vi "Start Menu.vi"(5 "Stats":string[][](table) caption="Result Set (from first statement with results)", 7 "Data Out":string[][](table) caption="Result Set (from first statement with results)", 8 "error in (no error)":errorcluster, 11 "Enum":enum16{"Initial Menu", "Final Menu"}(ring)) -> (0 "error out":errorcluster, 3 "Start/Stop":bool)   [LabVIEW 2021, in "Board Game.lvlib"]
uses:
  Board Game.lvlib
  <vilib>/Utility/miscctls.llb/LVRowAndColumnTypeDef.ctl
  Modules/Sound Manager/Typedefs/Sound Effects.ctl
  Utilities/Globales Snake.vi
  Modules/Sound Manager/Sound Manager.lvlib
panel:
  out "GAME STATS":bool
  in  "Player Name":string="user"
  out "INSTRUCTIONS":bool
  in  "Start Game":bool
  in  "GAME STATS":i32(listbox)
  out "LEADERBOARD":bool
  out "Instructions":bool
  in  "Play/stop":bool
  in  "Stop":bool
  in  "LEADERBOARD":i32(listbox)
  in  "Number of Bombs":i32=1
  in  "Play with Bombs":bool
  in  "Music:":u32(ring) items=["Music 1", "Music 2", "Music 3", "Music 4"]
  in  "Game Difficulty:":u32(ring)=150 items=["Easy"=750, "Hard"=500, "Extreme"=300, "Carlo Music"=150]
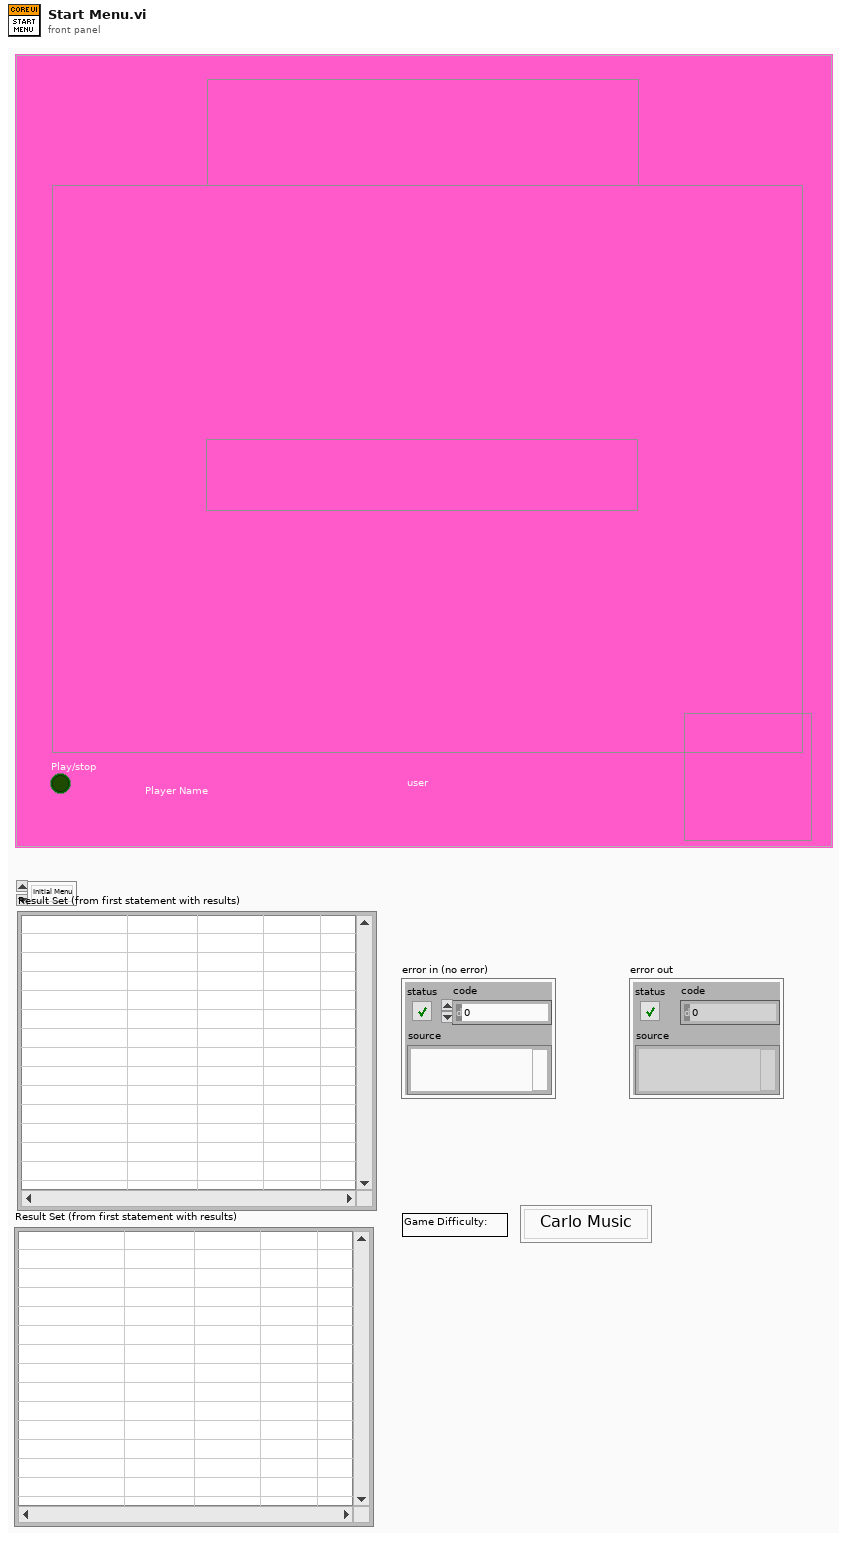
[diagram p1: front panel]
types:
  T1 = typedef "Sound Manager.lvlib/Sound Effects.ctl" = enum16{"Bomb In", "Bomb Out", "Bomb Touched", "Game Over", "Victory", "Eat", "10 Fruits", "Eat2", "Eat3", "Eat4", "MaxShield", "Shield", "10p", "Grape In", "Grape Out", "20p", "30p", "40p", "50p", "60p", "70p", "80p", "90p", "100p", "All shields cracked", "Mouse In", "Mouse Out", "Mouse Eaten", "Grape Eaten", "States Recover", "Broken Shield", "Bonus", "Happy Time", "explode", "Game over musica", "Back Music", "Shield Catch", "Evil lough", "Cricket In", "Cricket eaten", "Lets Go", "Jump1", "Jump2", "Jump3", "Unstoppable", "Troll Music", "winner", "menu"}
  T2 = typedef "LVRowAndColumnTypeDef.ctl" = cluster{"Row":i32, "Column":i32}
  T3 = cluster{"Music:":u32, "Game Difficulty:":u32, "Number of Bombs":i32}
  T4 = enum32{"Invalid", "Standard", "Closed", "Hidden", "Minimized", "Maximized"}
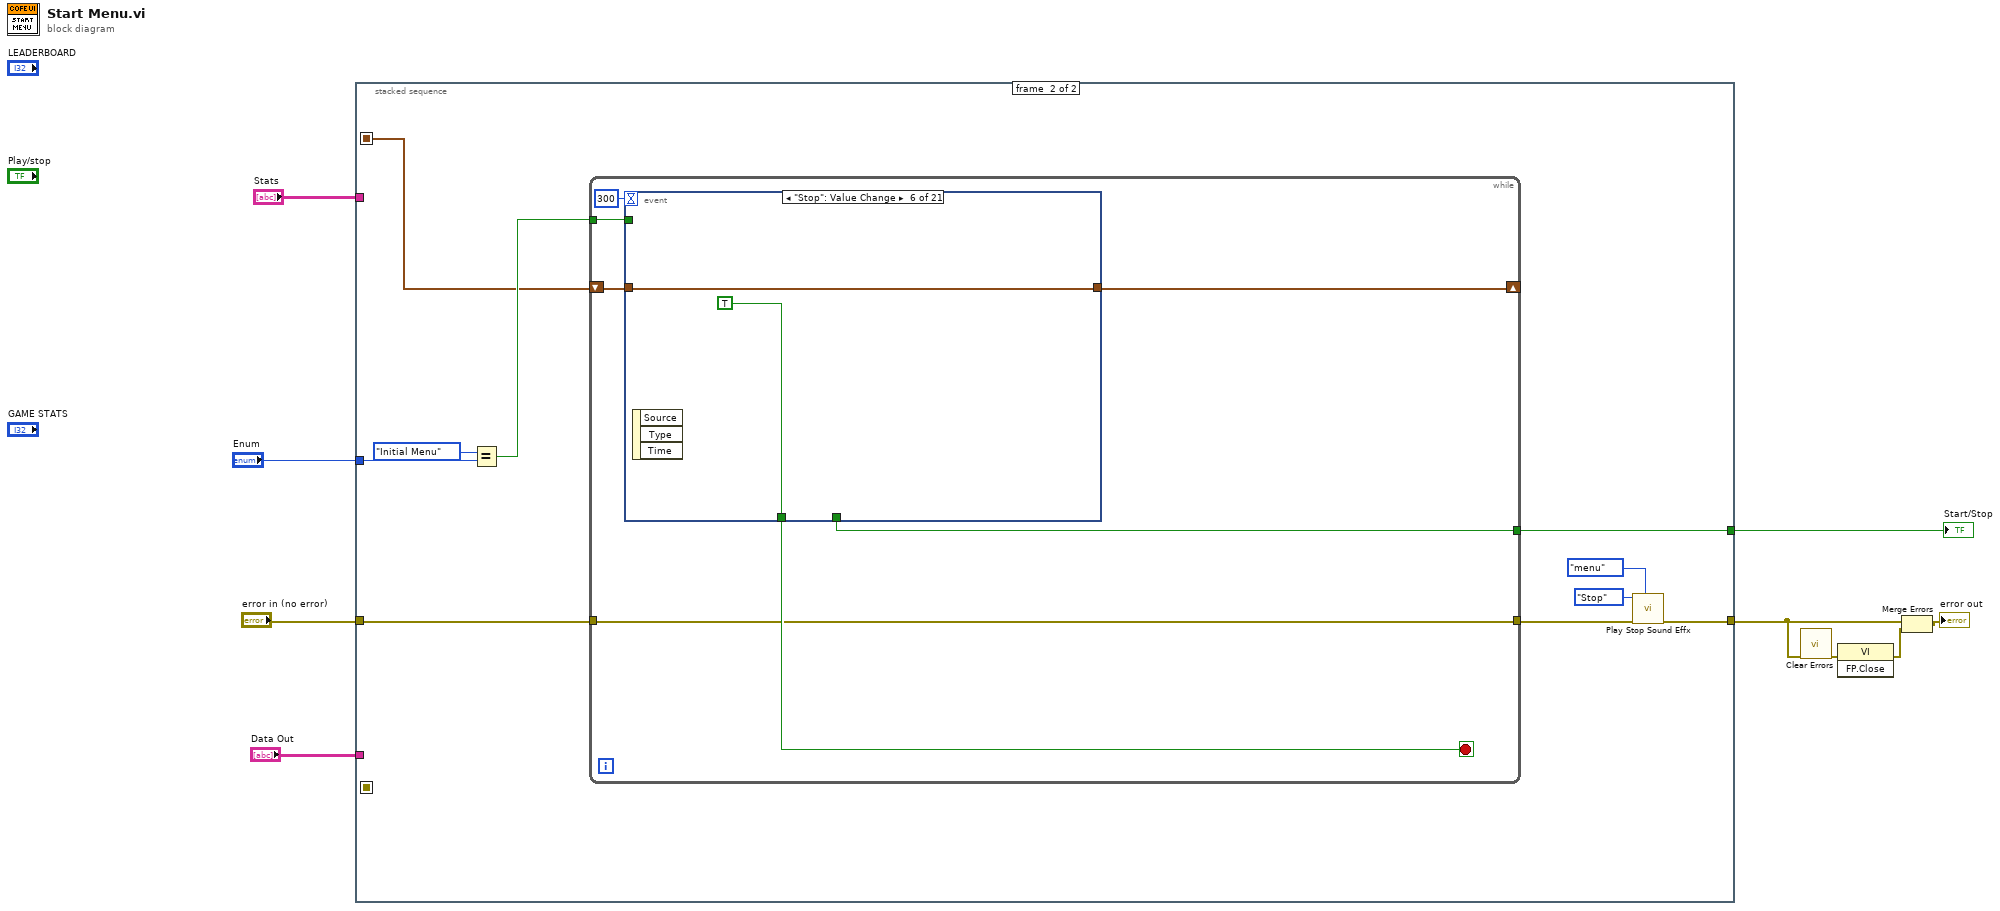
[diagram p0: block diagram]
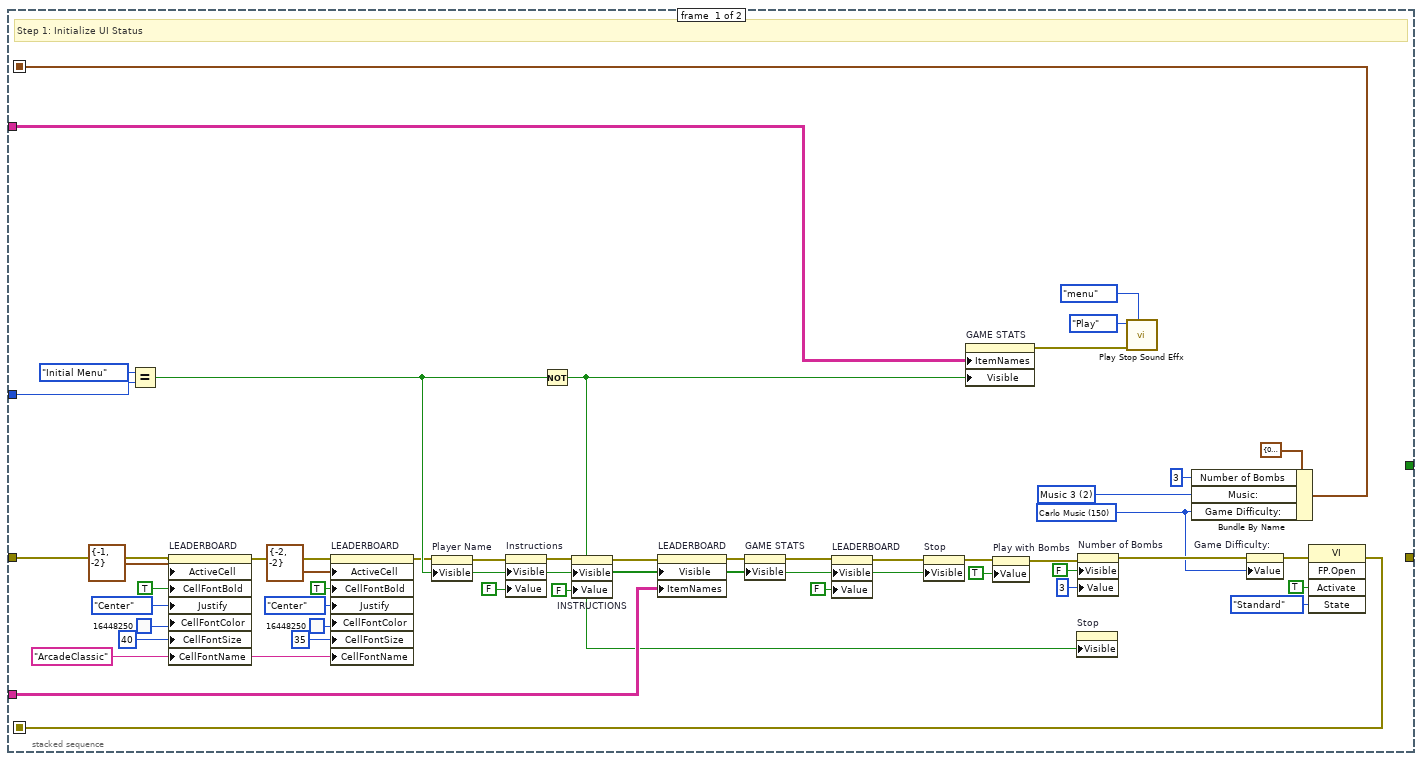
[diagram p2: hidden frame]
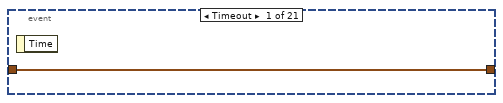
[diagram p3: hidden frame]
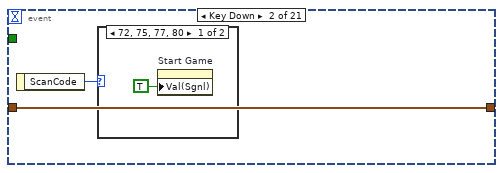
[diagram p4: hidden frame]
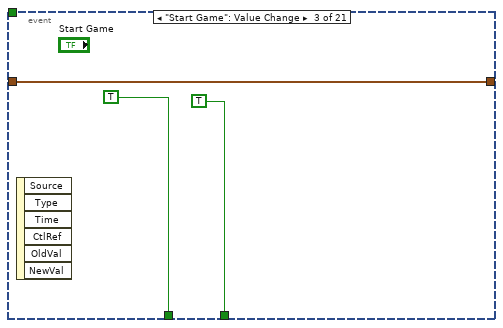
[diagram p6: hidden frame]
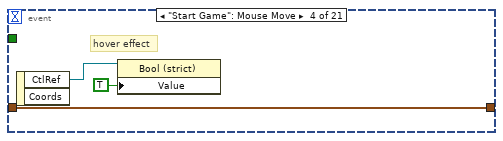
[diagram p7: hidden frame]
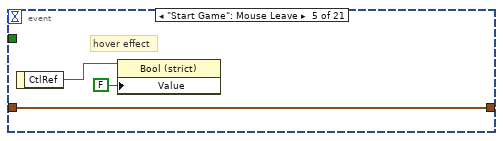
[diagram p8: hidden frame]
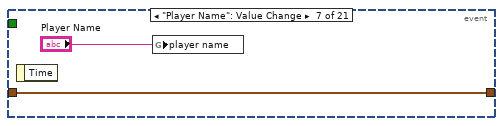
[diagram p9: hidden frame]
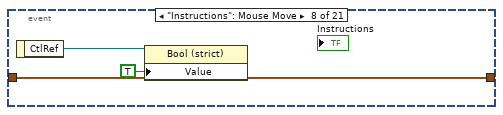
[diagram p10: hidden frame]
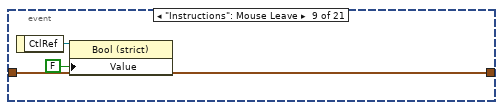
[diagram p11: hidden frame]
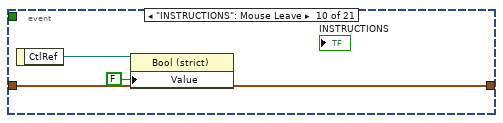
[diagram p12: hidden frame]
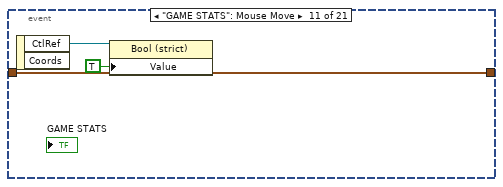
[diagram p13: hidden frame]
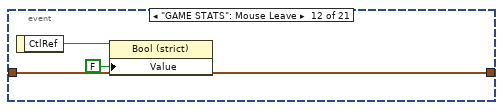
[diagram p14: hidden frame]
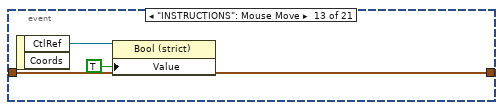
[diagram p15: hidden frame]
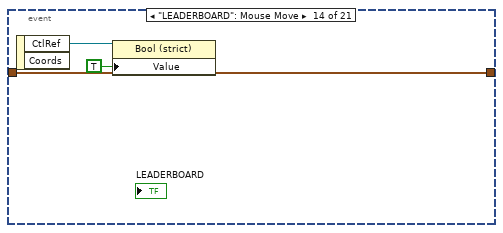
[diagram p16: hidden frame]
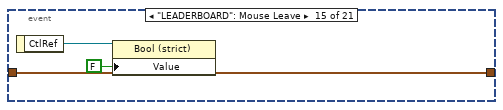
[diagram p17: hidden frame]
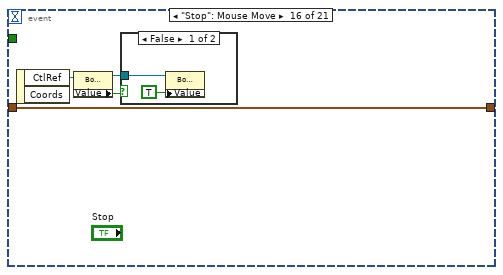
[diagram p18: hidden frame]
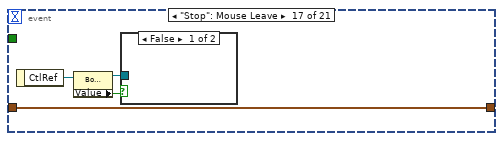
[diagram p20: hidden frame]
diagram:
  n1 = stacked-sequence {
    seq-local: [w32 _] -> [_ w63]
    seq-local: [w13 _] -> [_ _]
    tunnel: "Stats" -> [w14 _]
    tunnel: "Enum" -> [w31 w66]
    tunnel: "Data Out" -> [w21 _]
    tunnel: "error in (no error)" -> [w29 w62]
    tunnel: [_ w58] -> w4
    tunnel: [_ w57] -> w1
    frame #0 {
      w33 = "ArcadeClassic" ("Active Cell:Cell Font:Name")
      w47 = u32 150 items=["Easy"=750, "Hard"=500, "Extreme"=300, "Carlo Music"=150] ("Game Difficulty:")
      w48 = u32 2 items=["Music 1", "Music 2", "Music 3", "Music 4"] ("Music:")
      # "Step 1: Initialize UI Status"
      n2 = Equal?(x=enum16{"Initial Menu", "Final Menu"}."Initial Menu", y=w31) -> (x = y?=w28:bool)
      n3 = property on="LEADERBOARD" class="MCListbox (strict)"(error in=w29, "ActiveCell"=T2 {"Row"=-1, "Column"=-2} ("Active Cell:Active Cell"), "CellFontBold"=TRUE ("Active Cell:Cell Font:Bold"), "Justify"=enum16{"Left", "Center", "Right"}."Center" ("Active Cell:Cell Justification"), "CellFontColor"=u32 16448250 ("Active Cell:Cell Font:Color"), "CellFontSize"=u32 40 ("Active Cell:Cell Font:Size"), "CellFontName"=w33) -> (error out=w34:errorcluster)  [unwired: 1 in, 1 out]
      n4 = property on="LEADERBOARD" class="MCListbox (strict)"(error in=w34, "ActiveCell"=T2 {"Row"=-2, "Column"=-2} ("Active Cell:Active Cell"), "CellFontBold"=TRUE ("Active Cell:Cell Font:Bold"), "Justify"=enum16{"Left", "Center", "Right"}."Center" ("Active Cell:Cell Justification"), "CellFontColor"=u32 16448250 ("Active Cell:Cell Font:Color"), "CellFontSize"=u32 35 ("Active Cell:Cell Font:Size"), "CellFontName"=w33) -> (error out=w22:errorcluster)  [unwired: 1 in, 1 out]
      n5 = property on="Player Name" class="Str"(error in=w22, "Visible"=w28) -> (error out=w23:errorcluster)  [unwired: 1 in, 1 out]
      n6 = property on="Instructions" class="Bool (strict)"(error in=w23, "Visible"=w28, "Value"=FALSE ("Instructions")) -> (error out=w24:errorcluster)  [unwired: 1 in, 1 out]
      n7 = Not(x=w28) -> (.not. x?=w17:bool)
      n8 = property on="INSTRUCTIONS" class="Bool (strict)"(error in=w24, "Visible"=w28, "Value"=FALSE ("INSTRUCTIONS")) -> (error out=w25:errorcluster)  [unwired: 1 in, 1 out]
      n9 = property on="LEADERBOARD" class="MCListbox (strict)"(error in=w25, "Visible"=w17, "ItemNames"=w21) -> (error out=w20:errorcluster)  [unwired: 1 in, 1 out]
      n10 = property on="GAME STATS" class="MCListbox (strict)"(error in=w20, "Visible"=w17) -> (error out=w19:errorcluster)  [unwired: 1 in, 1 out]
      n11 = property on="LEADERBOARD" class="Bool (strict)"(error in=w19, "Visible"=w17, "Value"=FALSE ("Instructions")) -> (error out=w18:errorcluster)  [unwired: 1 in, 1 out]
      n12 = property on="Stop" class="Bool (strict)"(error in=w18, "Visible"=w17) -> (error out=w16:errorcluster)  [unwired: 1 in, 1 out]
      n13 = property on="GAME STATS" class="MCListbox (strict)"("ItemNames"=w14, "Visible"=w17) -> (error out=w12:errorcluster)  [unwired: 2 in, 1 out]
      n14 = property on="Play with Bombs" class="Bool (strict)"(error in=w16, "Value"=TRUE ("Play with Bombs")) -> (error out=w15:errorcluster)  [unwired: 1 in, 1 out]
      n15 = property on="Stop" class="Bool (strict)"("Visible"=w17) -> ()  [unwired: 2 in, 2 out]
      n16 = property on="Number of Bombs" class="DigNum (strict)"(error in=w15, "Visible"=FALSE, "Value"=3 ("Number of Bombs")) -> (error out=w53:errorcluster)  [unwired: 1 in, 1 out]
      n17 = call "Play Stop Sound Effx.vi"("Sound Effect"=Sound_Effects."menu", "Error In"=w12, "Function"=enum16{"Play", "Stop"}."Play") -> ()  [unwired: 8 in, 1 out]
      n18 = Bundle By Name(cluster=T3 {"Music:"=0, "Game Difficulty:"=150, "Number of Bombs"=1}, "Number of Bombs"=3, "Music:"=w48, "Game Difficulty:"=w47) -> (w32:T3)
      n19 = property on="Game Difficulty:" class="Ring (strict)"(error in=w53, "Value"=w47) -> (error out=w54:errorcluster)  [unwired: 1 in, 1 out]
      n20 = invoke class="VI" method="FP.Open"(error in=w54, "Activate"=TRUE ("Activate?"), "State"=T4."Standard") -> (error out=w13:errorcluster)  [unwired: 2 in, 4 out]
    }
    frame #1 {
      n21 = Equal?(x=enum16{"Initial Menu", "Final Menu"}."Initial Menu", y=w66) -> (x = y?=w64:bool)
      n22 = while {
        shift-right: [w71] -> _
        shift-left: w63 -> [w72]
        tunnel: w64 -> [w69]
        tunnel: w62 -> [w68]
        tunnel: [w68] -> w59
        tunnel: [w67] -> w57
        stop <- w73 stop-if-true
        n23 = event shown="[5] \"Stop\": Value Change" {
          selector: _ -> [_ _ _ _ _ _ _ _ _ _ _ _ _ _ _ _ _ _ _ _ _]
          dyn-events: _ -> [_ _ _ _ _ _ _ _ _ _ _ _ _ _ _ _ _ _ _ _ _]
          timeout: 300 -> [_ _ _ _ _ _ _ _ _ _ _ _ _ _ _ _ _ _ _ _ _]
          tunnel: [_ _ TRUE _ _ TRUE _ _ _ _ _ _ _ _ _ _ _ _ _ _ _] -> w73
          tunnel: w72 -> [w74 w76 w79 w83 w86 w87 w90 w93 w96 w99 w102 w105 w108 w111 w114 w118 w124 w129 w131 w134 w137]
          tunnel: [w74 w76 w79 w83 w86 w87 w90 w93 w96 w99 w102 w105 w108 w111 w114 w118 w124 w128 w132 w134 w136] -> w71
          tunnel: [_ _ TRUE _ _ _ _ _ _ _ _ _ _ _ _ _ _ _ _ _ _] -> w67
          tunnel: w69 -> [_ _ _ _ _ _ _ _ _ _ _ _ _ _ _ _ _ _ _ _ _]
          event Timeout {
            n24 = event-data() -> ()  [unwired: 1 in, 1 out]
          }
          event Key Down {
            n25 = event-data() -> ("ScanCode"=w75:i16)  [unwired: 1 in]
            n26 = case shown="72, 75, 77, 80" w75 {
              frame 72, 75, 77, 80 {
                n27 = property on="Start Game" class="Bool (strict)"("Val(Sgnl)"=TRUE ("Value (Signaling)")) -> ()  [unwired: 2 in, 2 out]
              }
              frame Default {
              }
            }
          }
          event "Start Game": Value Change {
            n28 = event-data() -> ()  [unwired: 1 in, 6 out]
          }
          event "Start Game": Mouse Move {
            # "hover effect"
            n29 = event-data() -> ("CtlRef"=w82:refnum<vi>)  [unwired: 1 in, 1 out]
            n30 = property class="Bool (strict)"(reference=w82, "Value"=TRUE) -> ()  [unwired: 1 in, 2 out]
          }
          event "Start Game": Mouse Leave {
            # "hover effect"
            n31 = event-data() -> ("CtlRef"=w85:refnum<vi>)  [unwired: 1 in]
            n32 = property class="Bool (strict)"(reference=w85, "Value"=FALSE) -> ()  [unwired: 1 in, 2 out]
          }
          event "Stop": Value Change {
            n33 = event-data() -> ()  [unwired: 1 in, 3 out]
          }
          event "Player Name": Value Change {
            n34 = event-data() -> ()  [unwired: 1 in, 1 out]
            n35 = global write "Globales Snake.vi" "player name"("Player Name") -> ()
          }
          event "Instructions": Mouse Move {
            n36 = event-data() -> ("CtlRef"=w92:refnum<vi>)  [unwired: 1 in]
            n37 = property class="Bool (strict)"(reference=w92, "Value"=TRUE) -> ()  [unwired: 1 in, 2 out]
          }
          event "Instructions": Mouse Leave {
            n38 = event-data() -> ("CtlRef"=w95:refnum<vi>)  [unwired: 1 in]
            n39 = property class="Bool (strict)"(reference=w95, "Value"=FALSE) -> ()  [unwired: 1 in, 2 out]
          }
          event "INSTRUCTIONS": Mouse Leave {
            n40 = event-data() -> ("CtlRef"=w98:refnum<vi>)  [unwired: 1 in]
            n41 = property class="Bool (strict)"(reference=w98, "Value"=FALSE) -> ()  [unwired: 1 in, 2 out]
          }
          event "GAME STATS": Mouse Move {
            n42 = event-data() -> ("CtlRef"=w101:refnum<vi>)  [unwired: 1 in, 1 out]
            n43 = property class="Bool (strict)"(reference=w101, "Value"=TRUE) -> ()  [unwired: 1 in, 2 out]
          }
          event "GAME STATS": Mouse Leave {
            n44 = event-data() -> ("CtlRef"=w104:refnum<vi>)  [unwired: 1 in]
            n45 = property class="Bool (strict)"(reference=w104, "Value"=FALSE) -> ()  [unwired: 1 in, 2 out]
          }
          event "INSTRUCTIONS": Mouse Move {
            n46 = event-data() -> ("CtlRef"=w107:refnum<vi>)  [unwired: 1 in, 1 out]
            n47 = property class="Bool (strict)"(reference=w107, "Value"=TRUE) -> ()  [unwired: 1 in, 2 out]
          }
          event "LEADERBOARD": Mouse Move {
            n48 = event-data() -> ("CtlRef"=w110:refnum<vi>)  [unwired: 1 in, 1 out]
            n49 = property class="Bool (strict)"(reference=w110, "Value"=TRUE) -> ()  [unwired: 1 in, 2 out]
          }
          event "LEADERBOARD": Mouse Leave {
            n50 = event-data() -> ("CtlRef"=w113:refnum<vi>)  [unwired: 1 in]
            n51 = property class="Bool (strict)"(reference=w113, "Value"=FALSE) -> ()  [unwired: 1 in, 2 out]
          }
          event "Stop": Mouse Move {
            n52 = event-data() -> ("CtlRef"=w117:refnum<vi>)  [unwired: 1 in, 1 out]
            n53 = property class="Bool (strict)"(reference=w117) -> (reference out=w115:refnum<vi>, "Value"=w116:bool)  [unwired: 1 in, 1 out]
            n54 = case shown="False" w116 {
              tunnel: w115 -> [w120 _]
              frame False {
                n55 = property class="Bool (strict)"(reference=w120, "Value"=TRUE) -> ()  [unwired: 1 in, 2 out]
              }
              frame True {
              }
            }
          }
          event "Stop": Mouse Leave {
            n56 = event-data() -> ("CtlRef"=w123:refnum<vi>)  [unwired: 1 in]
            n57 = property class="Bool (strict)"(reference=w123) -> (reference out=w121:refnum<vi>, "Value"=w122:bool)  [unwired: 1 in, 1 out]
            n58 = case shown="False" w122 {
              tunnel: w121 -> [_ w126]
              frame False {
              }
              frame True {
                n59 = property class="Bool (strict)"(reference=w126, "Value"=FALSE) -> ()  [unwired: 1 in, 2 out]
              }
            }
          }
          event "Game Difficulty:": Value Change {
            n60 = event-data() -> ("NewVal"=w127:u32)  [unwired: 1 in]
            n61 = Bundle By Name(cluster=w129, "Game Difficulty:"=w127) -> (w128:T3)
          }
          event "Music:": Value Change {
            n62 = event-data() -> ()  [unwired: 1 in, 6 out]
            n63 = Bundle By Name(cluster=w131, "Music:"="Music:") -> (w132:T3)
          }
          event "Play with Bombs": Value Change {
            n64 = event-data() -> ("NewVal"=w133:bool)  [unwired: 1 in]
            n65 = property on="Number of Bombs" class="DigNum (strict)"("Visible"=w133) -> ()  [unwired: 2 in, 2 out]
          }
          event "Number of Bombs": Value Change {
            n66 = event-data() -> ()  [unwired: 1 in, 6 out]
            n67 = Bundle By Name(cluster=w137, "Number of Bombs"="Number of Bombs") -> (w136:T3)
          }
        }
      }
      n68 = call "Play Stop Sound Effx.vi"("Sound Effect"=Sound_Effects."menu", "Error In"=w59, "Function"=enum16{"Play", "Stop"}."Stop") -> ("error in (no error)"=w58:errorcluster)  [unwired: 8 in]
    }
  }
  "Start/Stop" <- w1
  n69 = call <vilib>:"Clear Errors.vi"("error in (no error)"=w4) -> ("error out"=w5:errorcluster)  [unwired: 5 in, 1 out]
  n70 = invoke class="VI" method="FP.Close"(error in=w5) -> (error out=w3:errorcluster)  [unwired: 2 in, 2 out]
  n71 = Merge Errors(w4, w3) -> (→"error out":errorcluster)
